vi "DMSC.RegisterNewSystem.vi"(9 "myTasks":T1 {"processes"."restartMode" items=["UNKNOWN", "MANUAL", "ONCE", "ALWAYS", "KILL", "SHUTDOWN"]}, 11 "SDConnectionEvent":refnum<user-event>) -> ()   [LabVIEW 2014, in "DMSClient.lvlib"]
uses:
  DMSClient.lvlib
  DMSC.node_type.ctl
  DomainManagementUtils/DMSU.restart_mode.ctl
  DomainManagementUtils/DMSUtils.lvlib
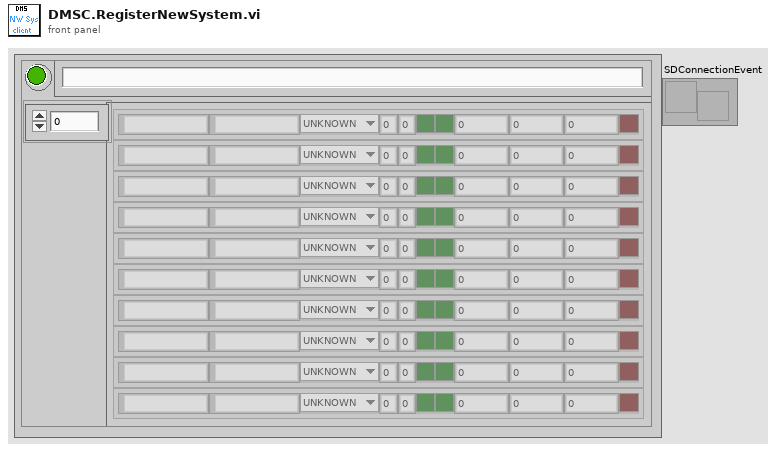
[diagram p1: front panel]
types:
  T1 = typedef "DMSClient.lvlib/DMSC.node_type.ctl" = cluster{"nodeName":string, "processes":cluster{"imageName":string, "argumentString":string, "restartMode":T2, "nOfRestart":i32, "resetRestartTimer":i32, "killOnExit":bool, "csSystem":bool, "PID":dbl, "PMem":dbl, "CPUTime":dbl, "startCnt":i32, "startTime":u32, "restartFailed":bool}[], "no link":bool}
  T2 = typedef "DMSUtils.lvlib/DMSU.restart_mode.ctl" = u16
  T3 = cluster{"imageName":string, "argumentString":string, "restartMode":T2, "nOfRestart":i32, "resetRestartTimer":i32, "killOnExit":bool, "csSystem":bool, "PID":dbl, "PMem":dbl, "CPUTime":dbl, "startCnt":i32, "startTime":u32, "restartFailed":bool}[]
  T4 = cluster{"Command":enum16{"NewSystem", "DestroySystem", "SDSystem"}, "argumentString":string}
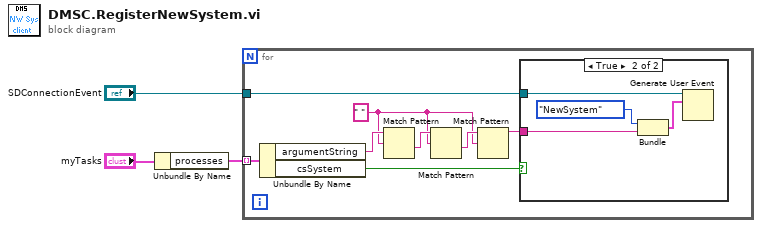
[diagram p0: block diagram]
diagram:
  n1 = Unbundle By Name("myTasks") -> ("processes"=w2:T3)
  n2 = for {
    tunnel: w2 -> [w7] mode=indexing
    tunnel: "SDConnectionEvent" -> [w4]
    w8 = " " ("regular expression")
    n3 = Unbundle By Name(w7) -> ("argumentString"=w11:string, "csSystem"=w6:bool)
    n4 = Match Pattern(string=w11, regular expression=w8) -> (after substring=w10:string)  [unwired: 1 in, 3 out]
    n5 = Match Pattern(string=w10, regular expression=w8) -> (after substring=w9:string)  [unwired: 1 in, 3 out]
    n6 = Match Pattern(string=w9, regular expression=w8) -> (before substring=w5:string)  [unwired: 1 in, 3 out]
    n7 = case shown="True" w6 {
      tunnel: w5 -> [_ w13]
      tunnel: w4 -> [_ w15]
      frame False {
      }
      frame True {
        n8 = Bundle("Command"=enum16{"NewSystem", "DestroySystem", "SDSystem"}."NewSystem", "argumentString"=w13) -> (w14:T4)  [unwired: 1 in]
        n9 = Generate User Event(user event=w15, event data cluster=w14) -> ()  [unwired: 2 in, 2 out]
      }
    }
  }
